vi "Deserialize Low Level Protocol Packet.vi"(0 "llp packet word":u8[](array[numeric])=[0, 0, 0, 0], 1 "reset":bool, 9 "input valid":bool, 12 "ready for output":bool=TRUE) -> (4 "tagged llp packet":T1={"tag"={"timestamp"={"valid"=FALSE, "count"=0.0, "id"=enum."SI0 LLP", "metadata"=0}, "size"={"bytes"=0.0, "valid"=FALSE}}, "llp packet"={"header"={"word count"=0, "ecc"=0.0, "vcx"=0.0, "data type"=0.0, "vc"=0.0}, "header valid"=FALSE, "payload"={"end of payload"=FALSE, "end of payload index"=0.0, "payload data"=[0, 0, 0, 0]}, "payload valid"=FALSE, "footer"={"crc"=0}, "footer valid"=FALSE, "end of packet"=FALSE}}, 10 "output valid":bool, 14 "ready for input":bool)   [LabVIEW 2020, in "GettingStarted_Common_148X_FPGA.lvlib"]
uses:
  GettingStarted_Common_148X_FPGA.lvlib
  <instrlib>/FlexRIO/CSI-2/v2/FPGA/Types/Tagged LLP Packet.ctl
  <instrlib>/FlexRIO/CSI-2/v2/FPGA/Types/FPGA LLP Packet Tag.ctl
  <instrlib>/FlexRIO/CSI-2/v2/FPGA/Types/FPGA LLP Packet Timestamp.ctl
  <instrlib>/FlexRIO/CSI-2/v2/FPGA/Types/Timestamp ID.ctl
  <instrlib>/FlexRIO/CSI-2/v2/FPGA/Types/FPGA LLP Packet Size.ctl
  <instrlib>/FlexRIO/CSI-2/v2/FPGA/Types/LLP Packet.ctl
  <instrlib>/FlexRIO/CSI-2/v2/FPGA/Types/LLP Packet Header.ctl
  <instrlib>/FlexRIO/CSI-2/v2/FPGA/Types/LLP Packet Payload.ctl
  <instrlib>/FlexRIO/CSI-2/v2/FPGA/Types/LLP Packet Footer.ctl
  <instrlib>/FlexRIO/CSI-2/v2/FPGA/Types/Deserialize LLP Packet State Data.ctl
  <instrlib>/FlexRIO/CSI-2/v2/FPGA/Types/Deserialize LLP Packet State.ctl
  <instrlib>/FlexRIO/CSI-2/v2/FPGA/Types/Raw Timestamp.ctl
  <instrlib>/_niInstr/Data Formatting/v1/FPGA/Private/Convert/U8 array to Boolean Array.vi
  <instrlib>/FlexRIO/CSI-2/v2/FPGA/NI CSI-2 API FPGA v2.lvlib
  <instrlib>/_niInstr/Data Formatting/v1/FPGA/niInstr Data Formatting v1 FPGA.lvlib
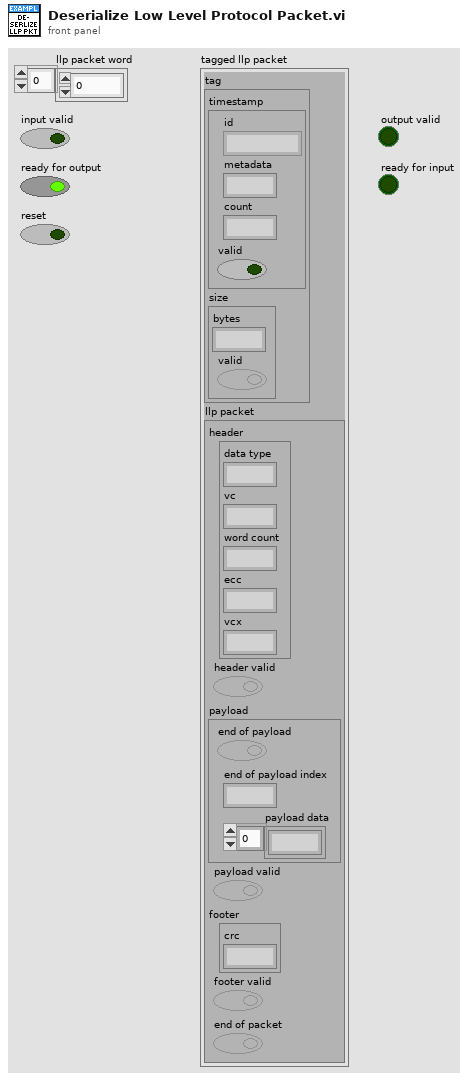
[diagram p1: front panel]
types:
  T1 = typedef "NI CSI-2 API FPGA v2.lvlib/Tagged LLP Packet.ctl" = cluster{"tag":T2, "llp packet":T6}
  T2 = typedef "NI CSI-2 API FPGA v2.lvlib/FPGA LLP Packet Tag.ctl" = cluster{"timestamp":T3, "size":T5}
  T3 = typedef "NI CSI-2 API FPGA v2.lvlib/FPGA LLP Packet Timestamp.ctl" = cluster{"valid":bool, "count":fxp<+,50,50>, "id":T4, "metadata":u8}
  T4 = typedef "NI CSI-2 API FPGA v2.lvlib/Timestamp ID.ctl" = enum8{"SI0 LLP", "SI1 LLP", "SI2 LLP", "SI3 LLP", "SI4 LLP", "SI5 LLP", "SI6 LLP", "SI7 LLP", "SO0 LLP", "SO1 LLP", "SO2 LLP", "SO3 LLP", "SO4 LLP", "SO5 LLP", "SO6 LLP", "SO7 LLP", "Ser0 GPIO Bank", "Ser1 GPIO Bank", "Ser2 GPIO Bank", "Ser3 GPIO Bank", "Ser4 GPIO Bank", "Ser5 GPIO Bank", "Ser6 GPIO Bank", "Ser7 GPIO Bank", "Des0 GPIO Bank", "Des1 GPIO Bank", "Des2 GPIO Bank", "Des3 GPIO Bank", "Des4 GPIO Bank", "Des5 GPIO Bank", "Des6 GPIO Bank", "Des7 GPIO Bank", "User0", "User1", "User2", "User3", "User4", "User5", "User6", "User7", "User8", "User9", "User10", "User11", "User12", "User13", "User14", "User15", "User16", "User17", "User18", "User19", "User20", "User21", "User22", "User23", "User24", "User25", "User26", "User27", "User28", "User29", "User30", "User31"}
  T5 = typedef "NI CSI-2 API FPGA v2.lvlib/FPGA LLP Packet Size.ctl" = cluster{"bytes":fxp<+,17,17>, "valid":bool}
  T6 = typedef "NI CSI-2 API FPGA v2.lvlib/LLP Packet.ctl" = cluster{"header":T7, "header valid":bool, "payload":T8, "payload valid":bool, "footer":T9, "footer valid":bool, "end of packet":bool}
  T7 = typedef "NI CSI-2 API FPGA v2.lvlib/LLP Packet Header.ctl" = cluster{"word count":u16, "ecc":fxp<+,6,6>, "vcx":fxp<+,2,2>, "data type":fxp<+,6,6>, "vc":fxp<+,2,2>}
  T8 = typedef "NI CSI-2 API FPGA v2.lvlib/LLP Packet Payload.ctl" = cluster{"end of payload":bool, "end of payload index":fxp<+,3,3>, "payload data":u8[]}
  T9 = typedef "NI CSI-2 API FPGA v2.lvlib/LLP Packet Footer.ctl" = cluster{"crc":u16}
  T10 = typedef "NI CSI-2 API FPGA v2.lvlib/Deserialize LLP Packet State.ctl" = enum8{"deserialize timestamp", "deserialize size and header", "deserialize payload"}
  T11 = typedef "NI CSI-2 API FPGA v2.lvlib/Deserialize LLP Packet State Data.ctl" = cluster{"llp packet cache":u8[], "llp packet cache size":fxp<+,4,4>, "timestamp":T3, "packet bytes remaining":fxp<+,17,17>, "state":T10}
  T12 = typedef "NI CSI-2 API FPGA v2.lvlib/Raw Timestamp.ctl" = cluster{"timestamp":u64, "valid":bool}
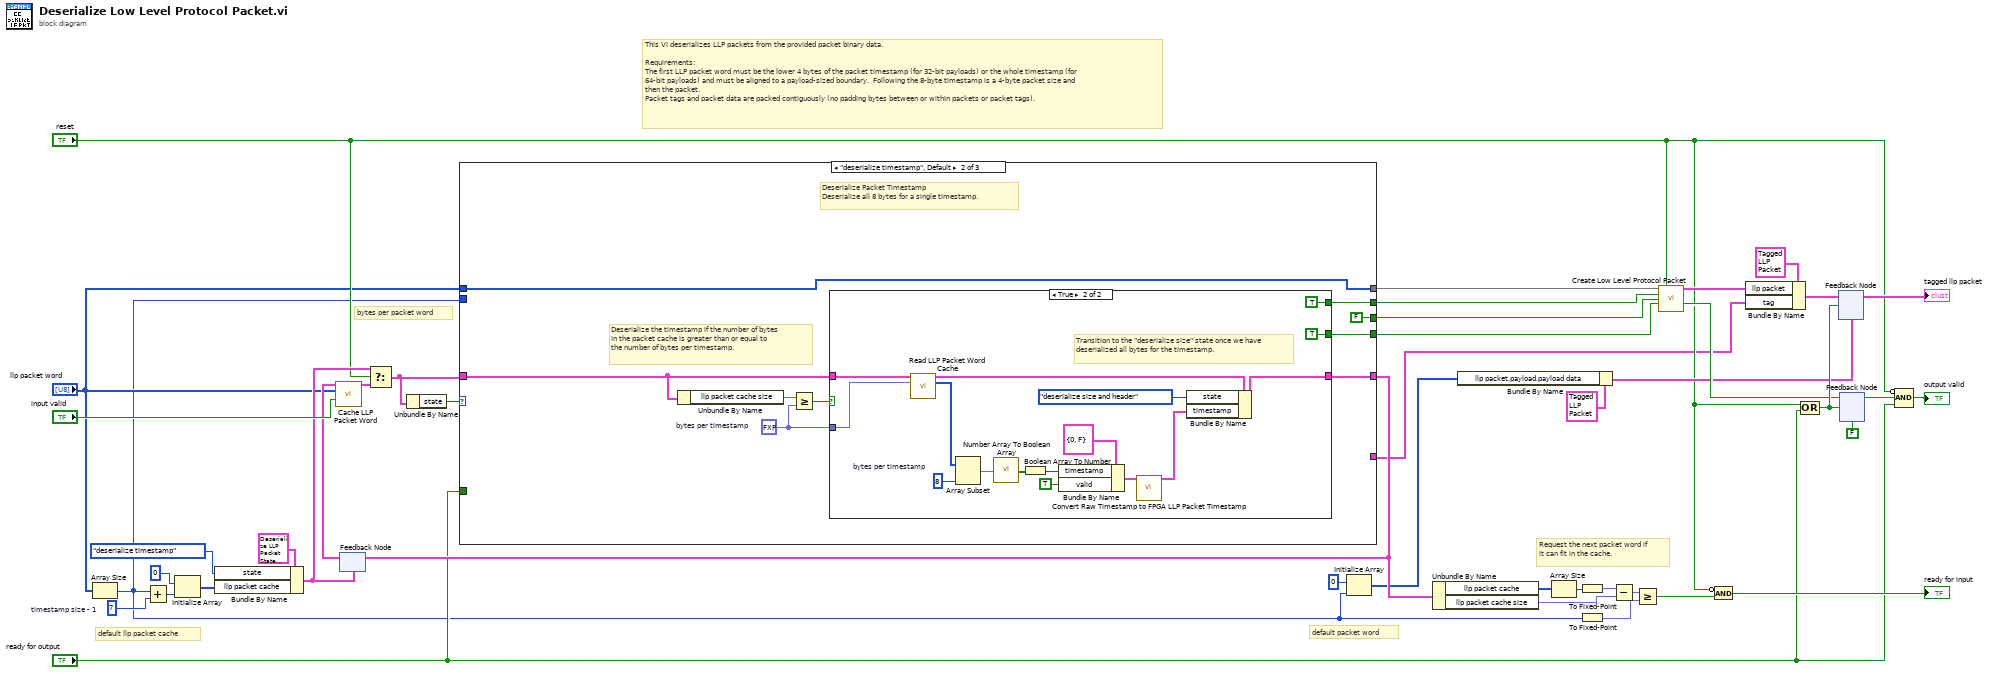
[diagram p0: block diagram]
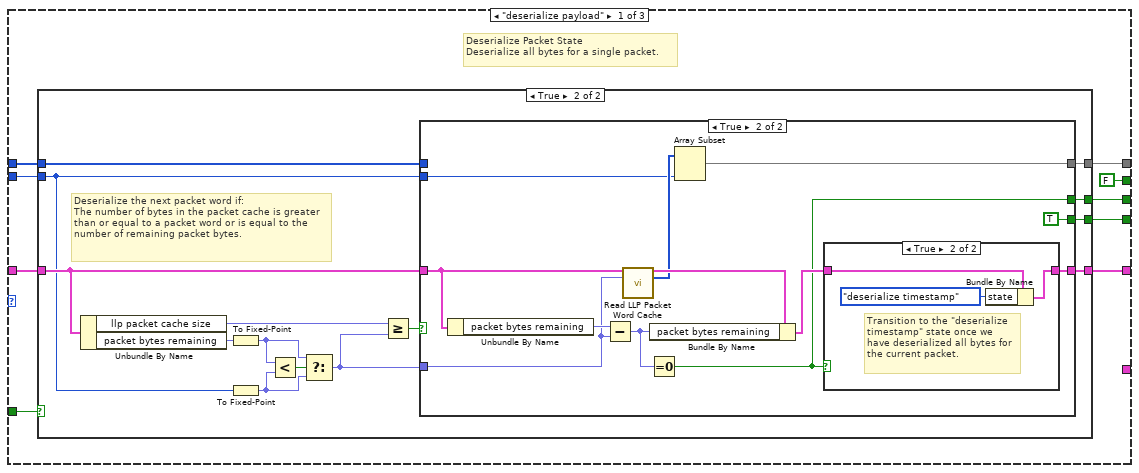
[diagram p2: hidden frame]
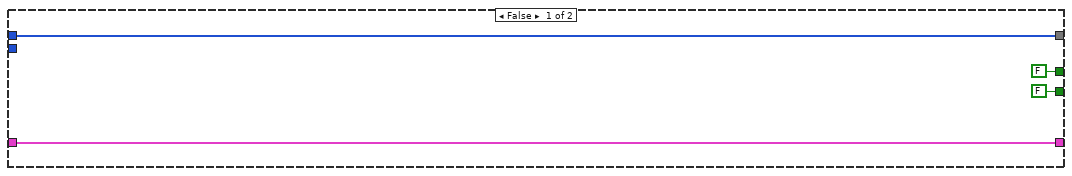
[diagram p3: hidden frame]
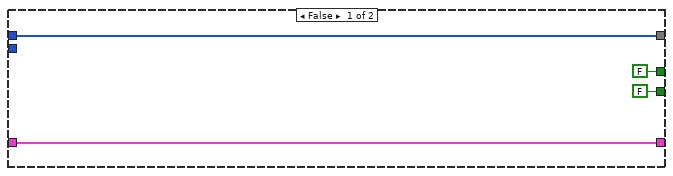
[diagram p4: hidden frame]
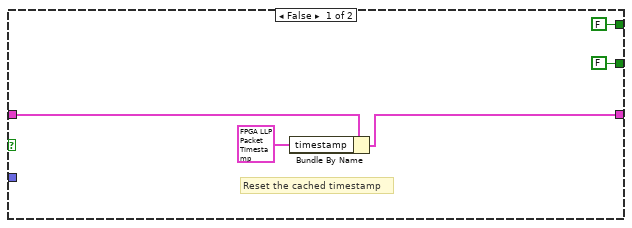
[diagram p6: hidden frame]
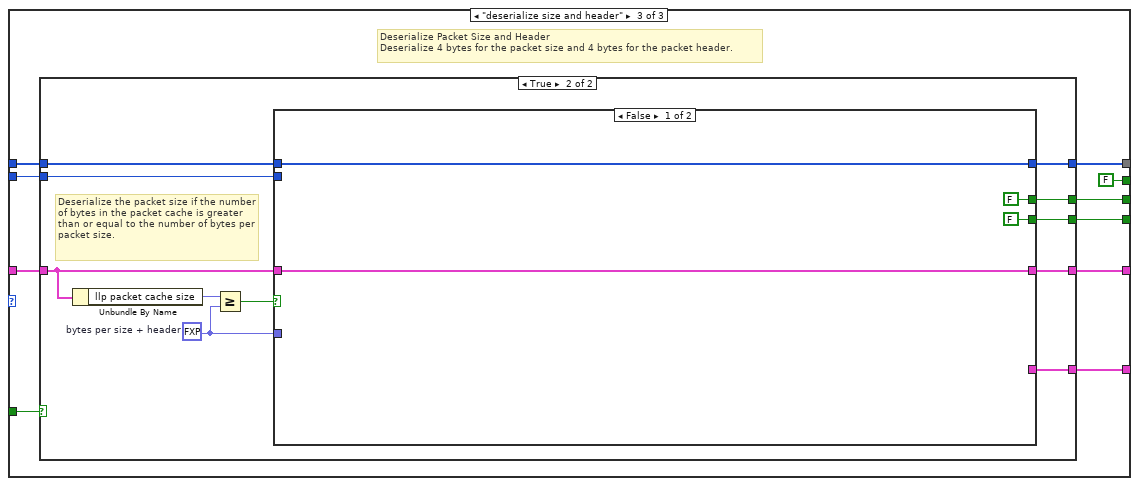
[diagram p7: hidden frame]
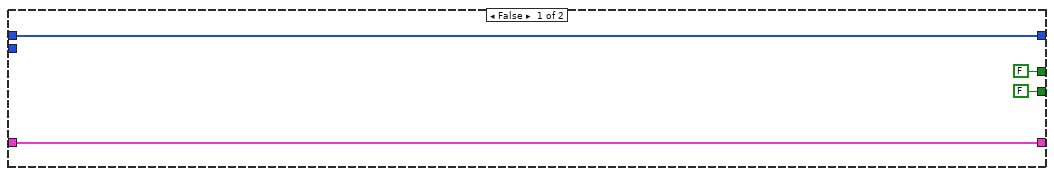
[diagram p8: hidden frame]
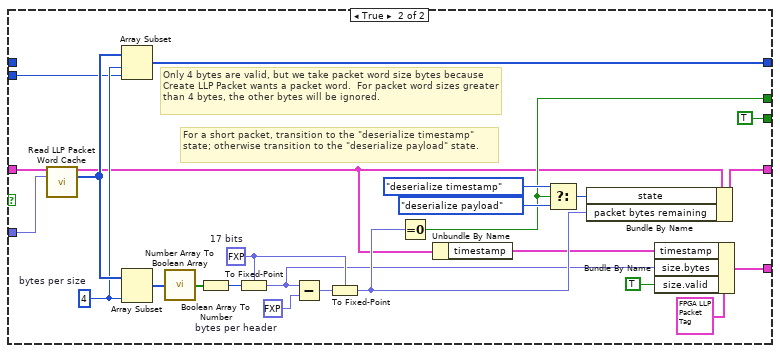
[diagram p9: hidden frame]
diagram:
  w21 = 7  # timestamp size - 1
  # "default llp packet cache"
  # "default packet word"
  # "bytes per packet word"
  # "Request the next packet word if it can fit in the cache."
  # "This VI deserializes LLP packets from the provided packet binary data.  \n\nRequirements:\nThe first LLP packet word must be the lower 4 bytes of the packet timestamp (for 32-bit payloads) or the whole timestamp (for 64-bit payloads) and must be aligned to a payload-sized boundary.  Following the 8-byte timestamp is a 4-byte packet size and then the packet.\nPacket tags and packet data are packed contiguously (no padding bytes between or within packets or packet tags)."
  n1 = Array Size(array="llp packet word") -> (size(s)=w8:i32)
  n2 = Add(x=w8, y=w21) -> (x+y=w20:i32)
  n3 = Initialize Array(u8 0 ("element"), w20) -> (w18:u8[])
  n4 = Bundle By Name(cluster=T11 {"llp packet cache"=[0, 0, 0, 0, 0, 0, 0, 0, 0, 0, 0], "llp packet cache size"=0.0, "timestamp"={"valid"=FALSE, "count"=0.0, "id"=enum."SI0 LLP", "metadata"=0}, "packet bytes remaining"=0.0, "state"=enum."deserialize payload"}, "state"=Deserialize_LLP_Packet_State."deserialize timestamp", "llp packet cache"=w18) -> (w26:T11)
  n5 = feedback #1(w26) -> (w30:T11)
  n6 = call "Cache LLP Packet Word.vi"("state in"=w30, "llp packet word"="llp packet word", "llp packet word valid"="input valid") -> ("state out"=w29:T11)  [unwired: 12 in]
  n7 = Select(t=w26, s="reset", f=w29) -> (s? t:f=w28:T11)
  n8 = Unbundle By Name(w28) -> ("state"=w40:T10)
  n9 = case shown="\"deserialize timestamp\", Default" w40 {
    tunnel: [FALSE ("start of transmission") w94 FALSE ("start of transmission")] -> w3
    tunnel: [w50 w92 w124] -> w4
    tunnel: [w48 w93 w128] -> w5
    tunnel: w28 -> [w51 w91 w130]
    tunnel: [w47 w99 w129] -> w27
    tunnel: "ready for output" -> [w49 _ w123]
    tunnel: [w46 FALSE ("output valid") w127] -> w2
    tunnel: "llp packet word" -> [w44 w92 w126]
    tunnel: w8 -> [w45 _ w122]
    tunnel: [_ _ w121] -> w1
    frame "deserialize payload" {
      # "Deserialize Packet State\nDeserialize all bytes for a single packet."
      n10 = case shown="True" w49 {
        tunnel: w51 -> [w55 w68]
        tunnel: [FALSE ("llp packet word valid") w69] -> w48
        tunnel: [w55 w65] -> w47
        tunnel: [w53 w70] -> w50
        tunnel: [FALSE w60] -> w46
        tunnel: w45 -> [_ w57]
        tunnel: w44 -> [w53 w59]
        frame False {
        }
        frame True {
          # "Deserialize the next packet word if:\nThe number of bytes in the packet cache is greater than or equal to a packet word or is equal to the number of remaining packet bytes."
          n11 = Unbundle By Name(w68) -> ("llp packet cache size"=w64:fxp<+,4,4>, "packet bytes remaining"=w63:fxp<+,17,17>)
          n12 = To Fixed-Point(number=w63) -> (fixed-point=w62:fxp<+,4,4>)  [unwired: 1 in]
          n13 = To Fixed-Point(number=w57) -> (fixed-point=w58:fxp<+,4,4>)  [unwired: 1 in]
          n14 = Less?(x=w62, y=w58) -> (x < y?=w67:bool)
          n15 = Select(t=w62, s=w67, f=w58) -> (s? t:f=w61:fxp<+,4,4>)
          n16 = Greater Or Equal?(x=w64, y=w61) -> (x >= y?=w66:bool)
          n17 = case shown="True" w66 {
            tunnel: [w71 w83] -> w70
            tunnel: [FALSE ("input valid") TRUE ("input valid")] -> w69
            tunnel: w68 -> [w74 w80]
            tunnel: [w74 w81] -> w65
            tunnel: w61 -> [_ w77]
            tunnel: [FALSE w76] -> w60
            tunnel: w57 -> [_ w75]
            tunnel: w59 -> [w71 _]
            frame False {
            }
            frame True {
              n18 = Unbundle By Name(w80) -> ("packet bytes remaining"=w85:fxp<+,17,17>)
              n19 = Subtract(x=w85, y=w77) -> (x-y=w84:fxp<+,17,17>)
              n20 = call "Read LLP Packet Word Cache.vi"("state in"=w80, "bytes to read"=w77) -> ("state out"=w79:T11, "cached bytes"=w78:u8[])  [unwired: 12 in]
              n21 = Equal To 0?(x=w84) -> (x = 0?=w76:bool)
              n22 = Bundle By Name(cluster=w79, "packet bytes remaining"=w84) -> (w82:T11)
              n23 = Array Subset(array=w78, length=w75) -> (w83:u8[])  [unwired: 1 in]
              n24 = case shown="True" w76 {
                tunnel: w82 -> [w87 w88]
                tunnel: [w87 w89] -> w81
                frame False {
                }
                frame True {
                  # "Transition to the \"deserialize timestamp\" state once we have deserialized all bytes for the current packet."
                  n25 = Bundle By Name(cluster=w88, "state"=Deserialize_LLP_Packet_State."deserialize timestamp") -> (w89:T11)
                }
              }
            }
          }
        }
      }
    }
    frame "deserialize timestamp", Default {
      w96 = fxp<+,4,4> 8.0  # bytes per timestamp
      # "Deserialize the timestamp if the number of bytes in the packet cache is greater than or equal to the number of bytes per timestamp."
      # "Deserialize Packet Timestamp\nDeserialize all 8 bytes for a single timestamp."
      n26 = Unbundle By Name(w91) -> ("llp packet cache size"=w97:fxp<+,4,4>)
      n27 = Greater Or Equal?(x=w97, y=w96) -> (x >= y?=w98:bool)
      n28 = case shown="True" w98 {
        tunnel: w91 -> [w102 w119]
        tunnel: [w101 w120] -> w99
        tunnel: w96 -> [_ w110]
        tunnel: [FALSE ("start of transmission") TRUE ("start of transmission")] -> w94
        tunnel: [FALSE ("output valid") TRUE ("output valid")] -> w93
        frame False {
          # "Reset the cached timestamp"
          n29 = Bundle By Name(cluster=w102, "timestamp"=T3 {"valid"=FALSE, "count"=0.0, "id"=enum."SI0 LLP", "metadata"=0}) -> (w101:T11)
        }
        frame True {
          w113 = 8  # bytes per timestamp
          # "Transition to the \"deserialize size\" state once we have deserialized all bytes for the timestamp."
          n30 = call "Read LLP Packet Word Cache.vi"("state in"=w119, "bytes to read"=w110) -> ("state out"=w118:T11, "cached bytes"=w112:u8[])  [unwired: 12 in]
          n31 = Array Subset(array=w112, length=w113) -> (w111:u8[])  [unwired: 1 in]
          n32 = call-poly <instrlib>:"Number Array To Boolean Array.vi"("data in"=w111) -> ("data out"=w117:bool[])  [unwired: 14 in]
          n33 = Boolean Array To Number(Boolean array=w117) -> (number=w116:u64)
          n34 = Bundle By Name(cluster=T12 {"timestamp"=0, "valid"=FALSE} ("raw timestamp"), "timestamp"=w116, "valid"=TRUE) -> (w109:T12)
          n35 = call <instrlib>:"Convert Raw Timestamp to FPGA LLP Packet Timestamp.vi"("raw timestamp"=w109) -> ("llp packet timestamp"=w107:T3)  [unwired: 14 in]
          n36 = Bundle By Name(cluster=w118, "state"=Deserialize_LLP_Packet_State."deserialize size and header", "timestamp"=w107) -> (w120:T11)
        }
      }
    }
    frame "deserialize size and header" {
      # "Deserialize Packet Size and Header\nDeserialize 4 bytes for the packet size and 4 bytes for the packet header."
      n37 = case shown="True" w123 {
        tunnel: w130 -> [w131 w145]
        tunnel: [w131 w144] -> w129
        tunnel: [FALSE ("output valid") w140] -> w128
        tunnel: [FALSE ("input valid") w139] -> w127
        tunnel: w126 -> [w134 w138]
        tunnel: [w134 w137] -> w124
        tunnel: w122 -> [_ w136]
        tunnel: [_ w135] -> w121
        frame False {
        }
        frame True {
          w141 = fxp<+,4,4> 8.0  # bytes per size + header
          # "Deserialize the packet size if the number of bytes in the packet cache is greater than or equal to the number of bytes per packet size."
          n38 = Unbundle By Name(w145) -> ("llp packet cache size"=w142:fxp<+,4,4>)
          n39 = Greater Or Equal?(x=w142, y=w141) -> (x >= y?=w143:bool)
          n40 = case shown="False" w143 {
            tunnel: w145 -> [w149 w173]
            tunnel: [w149 w174] -> w144
            tunnel: w141 -> [_ w170]
            tunnel: [FALSE ("output valid") TRUE ("output valid")] -> w140
            tunnel: [FALSE ("input valid") w160] -> w139
            tunnel: w138 -> [w146 _]
            tunnel: [w146 w157] -> w137
            tunnel: w136 -> [_ w156]
            tunnel: [_ w152] -> w135
            frame False {
            }
            frame True {
              w165 = fxp<+,17,17> 4.0  # bytes per header
              w166 = fxp<+,17,17> 0.0  # 17 bits
              w158 = 4  # bytes per size
              # "Only 4 bytes are valid, but we take packet word size bytes because Create LLP Packet wants a packet word.  For packet word sizes greater than 4 bytes, the other bytes will be ignored."
              # "For a short packet, transition to the \"deserialize timestamp\" state; otherwise transition to the \"deserialize payload\" state."
              n41 = call "Read LLP Packet Word Cache.vi"("state in"=w173, "bytes to read"=w170) -> ("state out"=w150:T11, "cached bytes"=w159:u8[])  [unwired: 12 in]
              n42 = Array Subset(array=w159, index=w158, length=w156) -> (w157:u8[])
              n43 = Array Subset(array=w159, length=w158) -> (w171:u8[])  [unwired: 1 in]
              n44 = call-poly <instrlib>:"Number Array To Boolean Array.vi"("data in"=w171) -> ("data out"=w172:bool[])  [unwired: 14 in]
              n45 = Boolean Array To Number(Boolean array=w172) -> (number=w169:u64)
              n46 = To Fixed-Point(fixed-point type=w166, number=w169) -> (fixed-point=w153:fxp<+,17,17>)
              n47 = Subtract(x=w153, y=w165) -> (x-y=w167:fxp<+/-,18,18>)
              n48 = To Fixed-Point(fixed-point type=w166, number=w167) -> (fixed-point=w161:fxp<+,17,17>)
              n49 = Equal To 0?(x=w161) -> (x = 0?=w160:bool)
              n50 = Unbundle By Name(w150) -> ("timestamp"=w151:T3)
              n51 = Select(t=Deserialize_LLP_Packet_State."deserialize timestamp" ("state"), s=w160, f=Deserialize_LLP_Packet_State."deserialize payload" ("state")) -> (s? t:f=w162:T10)
              n52 = Bundle By Name(cluster=w150, "state"=w162, "packet bytes remaining"=w161) -> (w174:T11)
              n53 = Bundle By Name(cluster=T2 {"timestamp"={"valid"=FALSE, "count"=0.0, "id"=enum."SI0 LLP", "metadata"=0}, "size"={"bytes"=0.0, "valid"=FALSE}} ("llp packet tag"), "timestamp"=w151, "size.bytes"=w153, "size.valid"=TRUE ("llp packet tag.size.valid")) -> (w152:T2)
            }
          }
        }
      }
    }
  }
  n54 = feedback-in #1(w27) -> ()
  n55 = Initialize Array(u8 0 ("element"), w8) -> (w7:u8[])
  n56 = Unbundle By Name(w27) -> ("llp packet cache"=w32:u8[], "llp packet cache size"=w35:fxp<+,4,4>)
  n57 = Bundle By Name(cluster=T1 {"tag"={"timestamp"={"valid"=FALSE, "count"=0.0, "id"=enum."SI0 LLP", "metadata"=0}, "size"={"bytes"=0.0, "valid"=FALSE}}, "llp packet"={"header"={"word count"=0, "ecc"=0.0, "vcx"=0.0, "data type"=0.0, "vc"=0.0}, "header valid"=FALSE, "payload"={"end of payload"=FALSE, "end of payload index"=0.0, "payload data"=[0, 0, 0, 0]}, "payload valid"=FALSE, "footer"={"crc"=0}, "footer valid"=FALSE, "end of packet"=FALSE}} ("llp packet"), "llp packet.payload.payload data"=w7) -> (w14:T1)
  n58 = Array Size(array=w32) -> (size(s)=w34:i32)
  n59 = To Fixed-Point(number=w34) -> (fixed-point=w33:fxp<+,4,4>)  [unwired: 1 in]
  n60 = To Fixed-Point(number=w8) -> (fixed-point=w16:fxp<+,4,4>)  [unwired: 1 in]
  n61 = Subtract(x=w33, y=w35) -> (x-y=w31:fxp<+,4,4>)
  n62 = Greater Or Equal?(x=w31, y=w16) -> (x >= y?=w6:bool)
  n63 = call <instrlib>:"Create Low Level Protocol Packet.vi"("data"=w4, "reset"="reset", "start of transmission"=w3, "end of transmission"=w2, "input valid"=w5) -> ("llp packet"=w22:T6, "output valid"=w23:bool)  [unwired: 9 in]
  n64 = Compound Arithmetic op=AND(invert "reset", w6) -> (→"ready for input":bool)
  n65 = Bundle By Name(cluster=T1 {"tag"={"timestamp"={"valid"=FALSE, "count"=0.0, "id"=enum."SI0 LLP", "metadata"=0}, "size"={"bytes"=0.0, "valid"=FALSE}}, "llp packet"={"header"={"word count"=0, "ecc"=0.0, "vcx"=0.0, "data type"=0.0, "vc"=0.0}, "header valid"=FALSE, "payload"={"end of payload"=FALSE, "end of payload index"=0.0, "payload data"=[0, 0, 0, 0]}, "payload valid"=FALSE, "footer"={"crc"=0}, "footer valid"=FALSE, "end of packet"=FALSE}} ("tagged llp packet"), "llp packet"=w22, "tag"=w1) -> (w24:T1)
  n66 = Compound Arithmetic op=OR("reset", "ready for output") -> (w38:bool)
  n67 = feedback #2(w14) -> (→"tagged llp packet":T1)
  n68 = feedback-in #2(w24, w38) -> ()
  n69 = feedback #3(FALSE ("output valid")) -> (w41:bool)
  n70 = feedback-in #3(w23, w38) -> ()
  n71 = Compound Arithmetic op=AND(invert "reset", w41, "ready for output") -> (→"output valid":bool)
